vi "show_match_items.vi"(9 "Match String":string, 11 "String Pool":refnum<vi>) -> (1 "Math Items Array":string[](array[string]))   [LabVIEW 2018]
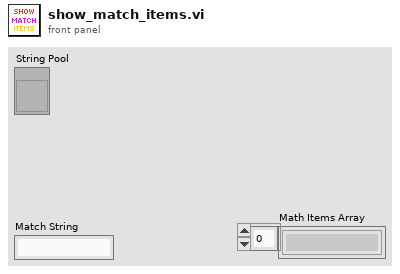
[diagram p1: front panel]
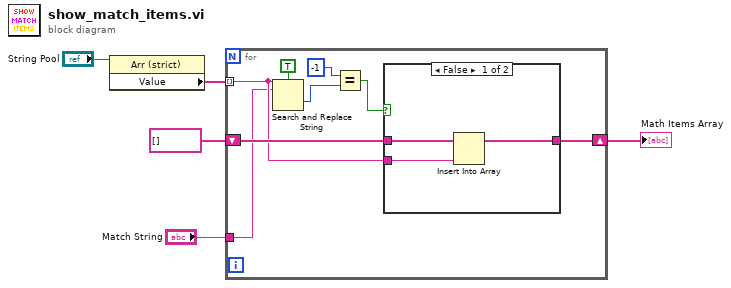
[diagram p0: block diagram]
diagram:
  n1 = property class="Arr (strict)"(reference="String Pool") -> ("Value"=w2:string[])  [unwired: 1 in, 2 out]
  n2 = for {
    tunnel: w2 -> [w7] mode=indexing
    shift-right: [w8] -> w1
    shift-left: string[] [] -> [w9]
    tunnel: "Match String" -> [w6]
    n3 = Search and Replace String(case sensitive?=TRUE ("ignore case? (F)"), input string=w7, search string=w6) -> (offset past replacement=w12:i32)  [unwired: 5 in, 3 out]
    n4 = Equal?(x=-1, y=w12) -> (x = y?=w10:bool)
    n5 = case shown="False" w10 {
      tunnel: w9 -> [w16 w17]
      tunnel: [w14 w17] -> w8
      tunnel: w7 -> [w15 _]
      frame False {
        n6 = Insert Into Array(array=w16, new element=w15) -> (w14:string[])  [unwired: 1 in]
      }
      frame True {
      }
    }
  }
  "Math Items Array" <- w1
